vi "Extract Array Elements.vi"(8 "error in (no error)":errorcluster, 11 "array reference in":T1 format="%.0x") -> (0 "error out":errorcluster, 1 "elements":T2[](array[typedef]), 2 "channel refnums":T1[](array[typedef]) format="%.0x", 3 "array reference out":T1 format="%.0x")   [LabVIEW 2018]
uses:
  <vilib>/NI Veristand/Custom Device API/Custom Device Item Ref.ctl
  APIs/Scripting API/TypeDefs/Array Element.ctl
  <vilib>/NI Veristand/Custom Device API/Custom Device API.lvlib
  APIs/Scripting API/Instrument Addon Scripting API.lvlib
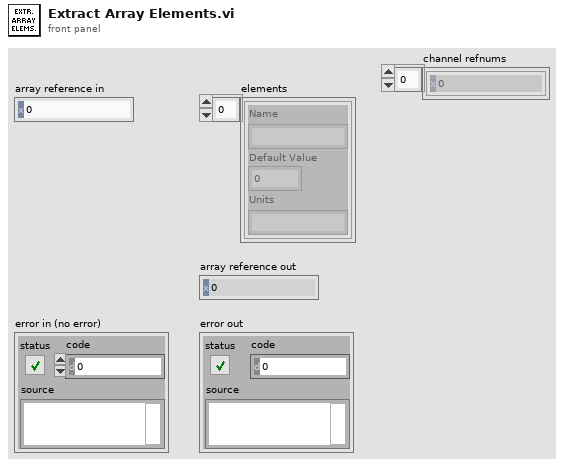
[diagram p1: front panel]
types:
  T1 = typedef "Custom Device API.lvlib/Custom Device Item Ref.ctl" = u64
  T2 = typedef "Instrument Addon Scripting API.lvlib/Array Element.ctl" = cluster{"Name":string, "Default Value":dbl, "Units":string}
  T3 = typedef "Custom Device API.lvlib/Custom Device Channel.ctl" = cluster{"Type":T4, "Units":string, "Default Value":dbl, "Faultable":bool, "Scalable":bool}
  T4 = typedef "Custom Device API.lvlib/Custom Device Channel Type.ctl" = enum16{"Input", "Output"}
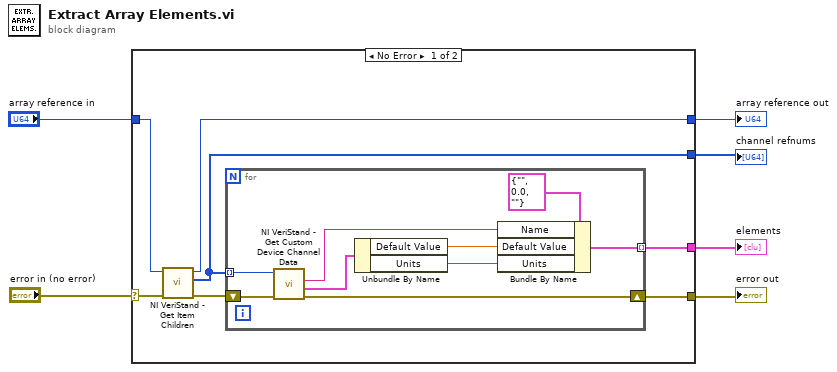
[diagram p0: block diagram]
diagram:
  n1 = case shown="No Error" "error in (no error)" {
    selector: "error in (no error)" -> [w8 w23]
    tunnel: [w13 w24] -> w6
    tunnel: [w12 w23] -> w5
    tunnel: "array reference in" -> [w10 w24]
    tunnel: [w9 _] -> w3
    tunnel: [w7 _] -> w1
    frame No Error {
      n2 = call <vilib>:"NI VeriStand - Get Item Children.vi"("error in (no error)"=w8, "Item Ref in"=w10) -> ("error out"=w11:errorcluster, "Child Refs"=w7:T1[], "Item Ref out"=w13:T1)  [unwired: 6 in, 1 out]
      n3 = for {
        tunnel: w7 -> [w20] mode=indexing
        shift-right: [w21] -> w12
        shift-left: w11 -> [w22]
        tunnel: [w18] -> w9 mode=indexing
        n4 = call <vilib>:"NI VeriStand - Get Custom Device Channel Data.vi"("error in (no error)"=w22, "Channel Ref in"=w20) -> ("error out"=w21:errorcluster, "Channel"=w16:T3, "Channel Name"=w17:string)  [unwired: 4 in, 3 out]
        n5 = Unbundle By Name(w16) -> ("Default Value"=w15:dbl, "Units"=w14:string)
        n6 = Bundle By Name(cluster=T2 {"Name"="", "Default Value"=0.0, "Units"=""} ("Array Element"), "Name"=w17, "Default Value"=w15, "Units"=w14) -> (w18:T2)
      }
    }
    frame Error {
    }
  }
  "array reference out" <- w6
  "elements" <- w3
  "error out" <- w5
  "channel refnums" <- w1
